vi "H5Lget_info_by_idx.vi"(5 "Order":T1 items=["H5_ITER_UNKNOWN"=-1, "H5_ITER_INC"=0, "H5_ITER_DEC"=1], 6 "lapl_id":T6, 7 "Index Field":T2 items=["H5_INDEX_UNKNOWN"=-1, "H5_INDEX_NAME"=0, "H5_INDEX_CRT_ORDER"=1], 8 "error in (no error)":errorcluster, 9 "Index":u64, 10 "Group Name":string=".", 11 "Location Ref":T6) -> (0 "error out":errorcluster, 2 "H5L_info_t":T3 {"cset" items=["H5T_CSET_ERROR"=-1, "H5T_CSET_ASCII"=0, "H5T_CSET_UTF8"=1]; "type" items=["H5L_TYPE_ERROR"=-1, "H5L_TYPE_HARD"=0, "H5L_TYPE_SOFT"=1, "H5L_TYPE_EXTERNAL"=64, "H5L_TYPE_MAX"=255]}, 3 "Location Ref out":T6)   [LabVIEW 2017]
doc: "Retrieves metadata for a link in a group, according to the order \n within a field or index."
uses:
  <vilib>/UPVI/lvhdf5/library.llb/HDF5 Ref.ctl
  <vilib>/UPVI/lvhdf5/link.llb/H5L_info_t.ctl
  <vilib>/UPVI/lvhdf5/link.llb/H5L_type_t.ctl
  <vilib>/UPVI/lvhdf5/datatype.llb/H5T_cset_t.ctl
  <vilib>/UPVI/lvhdf5/library.llb/H5_index_t.ctl
  <vilib>/UPVI/lvhdf5/library.llb/H5_iter_order_t.ctl
  <vilib>/UPVI/lvhdf5/h5helper.dll
  <vilib>/UPVI/lvhdf5/hdf5.dll
panel:
  # "LVHDF5 Toolkit\nCopyright (c) 2005-2013 by Jason D. Sommerville\nCopyright (c) 2014-2015 by UPVI, LLC.\n\nThis use and distribution of this file is governed by the terms found in \nLICENSE.txt distributed with this toolkit and installed at\n <user.lib>\\_lvhdf5\\LICENSE.txt"
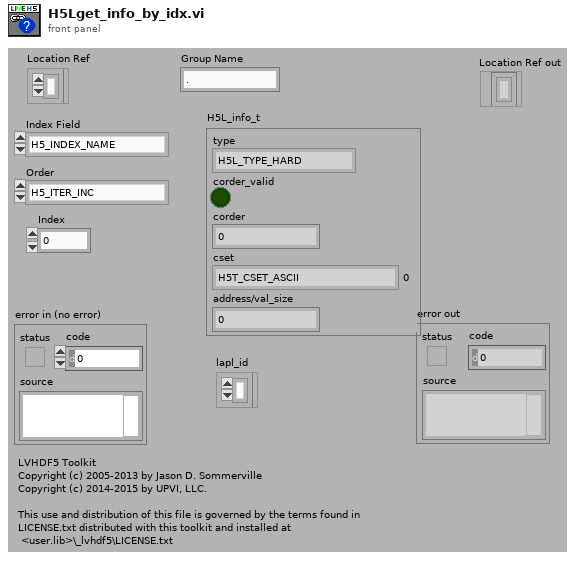
[diagram p1: front panel]
types:
  T1 = typedef "H5_iter_order_t.ctl" = i32
  T2 = typedef "H5_index_t.ctl" = i32
  T3 = typedef "H5L_info_t.ctl" = cluster{"type":T4, "corder_valid":bool, "corder":i64, "cset":T5, "address/val_size":u64}
  T4 = typedef "H5L_type_t.ctl" = i32
  T5 = typedef "H5T_cset_t.ctl" = i32
  T6 = typedef "HDF5 Ref.ctl" = refnum<k1>
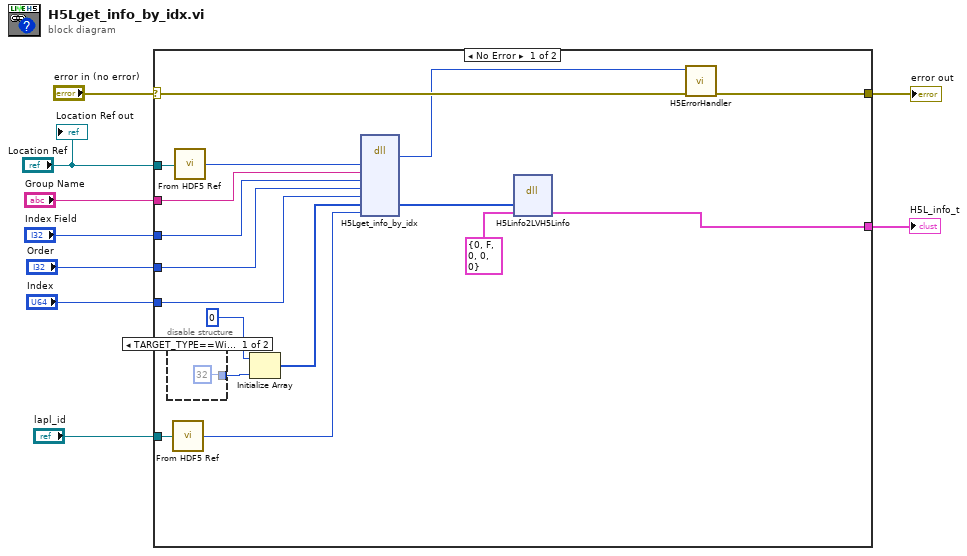
[diagram p0: block diagram]
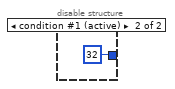
[diagram p2: hidden frame]
diagram:
  n1 = case shown="No Error" "error in (no error)" {
    selector: "error in (no error)" -> [w26 w29]
    tunnel: [w25 w29] -> w8
    tunnel: "lapl_id" -> [w24 _]
    tunnel: "Location Ref" -> [w21 _]
    tunnel: "Group Name" -> [w19 _]
    tunnel: [w13 _] -> w4
    tunnel: "Index Field" -> [w12 _]
    tunnel: "Order" -> [w11 _]
    tunnel: "Index" -> [w10 _]
    frame No Error {
      n2 = disable-structure shown="TARGET_TYPE==Windows&&TARGET_BITNESS==32, default" {
        disable-tunnel: [32 32] -> w18
        frame condition #0 {
        }
        frame condition #1 (active) {
        }
      }
      n3 = call <vilib>:"From HDF5 Ref.vi"("HDF5 Ref"=w24) -> ("I32"=w23:i32)
      n4 = call <vilib>:"From HDF5 Ref.vi"("HDF5 Ref"=w21) -> ("I32"=w20:i32)
      n5 = Initialize Array(u8 0, w18) -> (w16:u8[])
      n6 = dll-call lib="C:/Program Files/National Instruments/LabVIEW 2017/vi.lib/UPVI/lvhdf5/hdf5.dll" fn="H5Lget_info_by_idx" label="H5Lget_info"("loc_id"=w20, "group_name"=w19, "index_field"=w12, "order"=w11, "n"=w10, "link_buff"=w16, "lapl_id"=w23) -> ("return type"=w22:i32, "link_buff"=w15:u8[])  [unwired: 9 in, 2 out]
      n7 = dll-call lib="C:/Program Files/National Instruments/LabVIEW 2017/vi.lib/UPVI/lvhdf5/h5helper.dll" fn="H5Linfo2LVH5Linfo"("H5Linfo"=w15, "LVH5Linfo"=T3 {"type"=0, "corder_valid"=FALSE, "corder"=0, "cset"=0, "address/val_size"=0} ("H5L_info_t")) -> ("LVH5Linfo"=w13:T3)  [unwired: 5 in, 2 out]
      n8 = call <vilib>:"H5ErrorHandler.vi"("error in (no error)"=w26, "herr_t"=w22) -> ("error out"=w25:errorcluster)  [unwired: 3 in, 4 out]
    }
    frame Error {
    }
  }
  "error out" <- w8
  "H5L_info_t" <- w4
  "Location Ref out" <- "Location Ref"
